vi "setPathAndType.vi"(8 "error in (no error)":errorcluster, 9 "fileType":T1, 10 "Path":path, 11 "reference in":refnum<class "excelFile.lvclass">) -> (0 "error out":errorcluster, 3 "reference out":refnum<class "excelFile.lvclass">)   [LabVIEW 2015, in "excelFile.lvclass"]
uses:
  excelFile.lvclass
  fileType.ctl
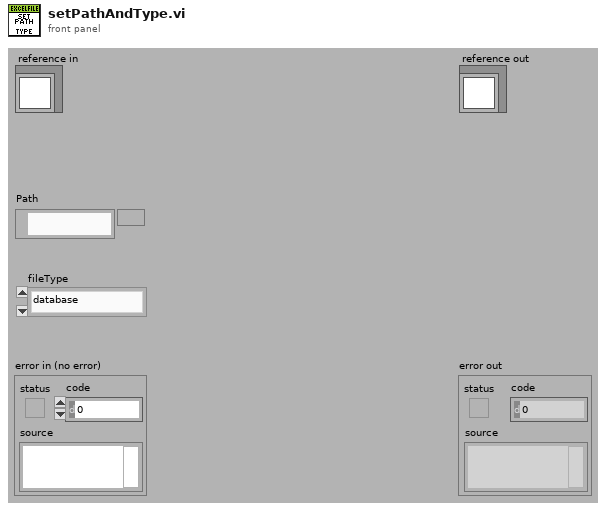
[diagram p1: front panel]
types:
  T1 = typedef "excelFile.lvclass/fileType.ctl" = enum16{"database", "CosmedTest"}
  T2 = typedef "excelFile.lvclass/ObjectAttributesRef.ctl" = refnum<data-value>
  T3 = typedef "excelFile.lvclass/ObjectAttributes.ctl" = cluster{"MyAttribute":dbl, "path":string, "Refnum Excel":cluster{"Excel._Application":refnum<k7>, "Workbooks":refnum<k7>, "Open":refnum<k7>}, "data":string[][][], "fileType":T1, "sheetName":string[]}
  T4 = typedef "excelFile.lvclass/ClassAttributesRef.ctl" = refnum<data-value>
  T5 = typedef "excelFile.lvclass/ClassAttributes.ctl" = cluster{"Dummy":bool, "excelFile_refs":refnum<class "excelFile.lvclass">[]}
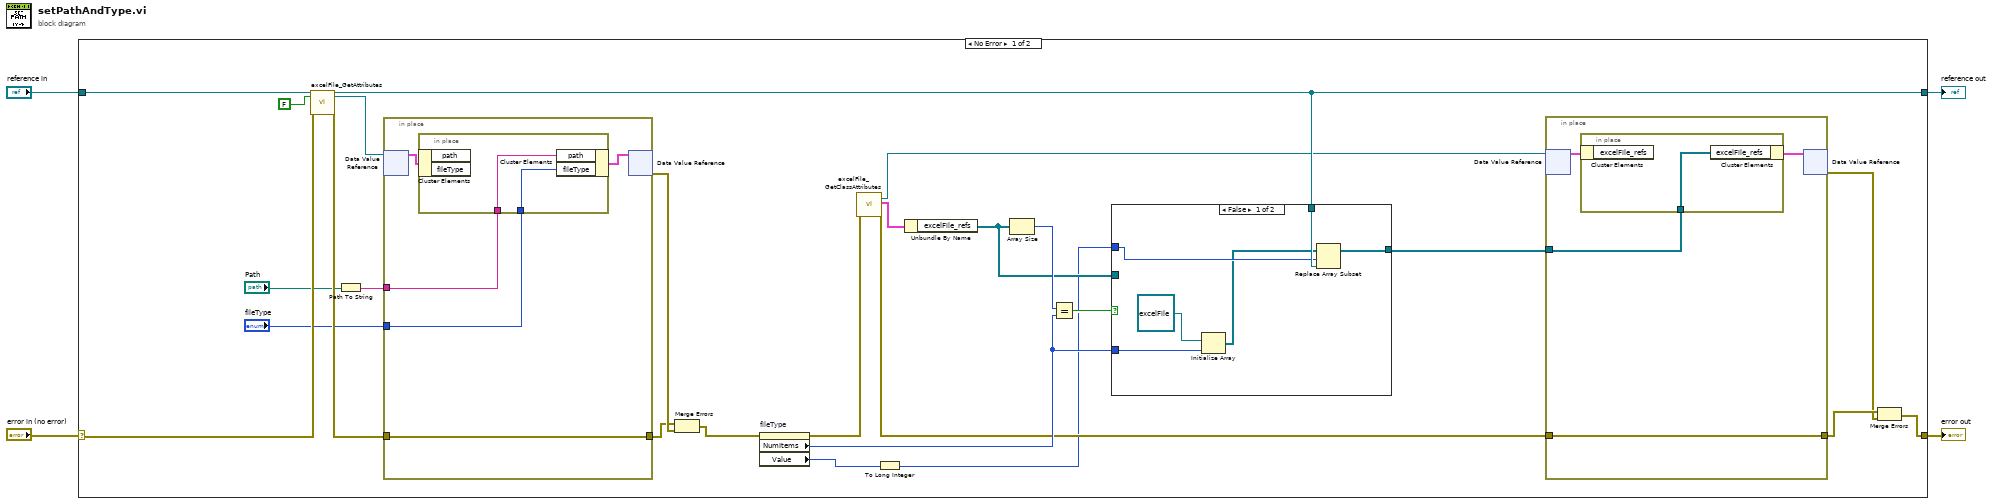
[diagram p0: block diagram]
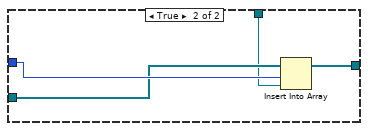
[diagram p2: hidden frame]
diagram:
  n1 = case shown="No Error" "error in (no error)" {
    selector: "error in (no error)" -> [w26 w54]
    tunnel: [w6 w54] -> w3
    tunnel: [w14 w53] -> w1
    tunnel: "reference in" -> [w28 w53]
    frame No Error {
      n2 = call "excelFile_GetAttributes.vi"("reference in"=w28, "return data? (T)"=FALSE, "error in (no error)"=w26) -> ("reference out"=w14:refnum<class "excelFile.lvclass">, "attributes ref"=w24:T2, "error out"=w25:errorcluster)  [unwired: 13 in, 1 out]
      n3 = Path To String(path="Path") -> (string=w22:string)
      n4 = in-place {
        in-place-border: w25 -> [w48]
        in-place-border: [w48] -> w29
        in-place-border: w22 -> [w47]
        in-place-border: "fileType" -> [w46]
        n5 = in-place-dvr #1(w24) -> (w49:T3)  [unwired: 1 out]
        n6 = in-place {
          in-place-border: w47 -> [w52]
          in-place-border: w46 -> [w51]
          n7 = in-place-cluster #2(w49) -> ()  [unwired: 2 out]
          n8 = in-place-cluster #2("path"=w52, "fileType"=w51) -> (w50:T3)
        }
        n9 = in-place-dvr #1(w50) -> (w30:errorcluster)  [unwired: 1 out]
      }
      n10 = Merge Errors(w29, w30) -> (w21:errorcluster)
      n11 = property on="fileType" class="Enum (strict)"(error in=w21) -> (error out=w20:errorcluster, "NumItems"=w15:u32, "Value"=w9:T1)  [unwired: 1 in, 1 out]
      n12 = call "excelFile_GetClassAttributes.vi"("error in (no error)"=w20) -> ("class attributes ref"=w11:T4, "class attributes"=w19:T5, "error out"=w12:errorcluster)  [unwired: 15 in, 1 out]
      n13 = To Long Integer(number=w9) -> (32bit integer=w8:i32)
      n14 = Unbundle By Name(w19) -> ("excelFile_refs"=w13:refnum<class "excelFile.lvclass">[])
      n15 = Array Size(array=w13) -> (size(s)=w18:i32)
      n16 = Equal?(x=w18, y=w15) -> (x = y?=w17:bool)
      n17 = case shown="False" w17 {
        tunnel: w8 -> [w38 w45]
        tunnel: w15 -> [w40 _]
        tunnel: w14 -> [w39 w43]
        tunnel: w13 -> [_ w44]
        tunnel: [w36 w42] -> w10
        frame False {
          n18 = Initialize Array(refnum<class "excelFile.lvclass"> refnum ("excelFile.lvclass"), w40) -> (w37:refnum<class "excelFile.lvclass">[])
          n19 = Replace Array Subset(array=w37, new element=w39, index=w38) -> (w36:refnum<class "excelFile.lvclass">[])
        }
        frame True {
          n20 = Insert Into Array(array=w44, index=w45, new element=w43) -> (w42:refnum<class "excelFile.lvclass">[])
        }
      }
      n21 = in-place {
        in-place-border: w12 -> [w32]
        in-place-border: [w32] -> w7
        in-place-border: w10 -> [w31]
        n22 = in-place-dvr #3(w11) -> (w33:T5)  [unwired: 1 out]
        n23 = in-place {
          in-place-border: w31 -> [w35]
          n24 = in-place-cluster #4(w33) -> ()  [unwired: 1 out]
          n25 = in-place-cluster #4("excelFile_refs"=w35) -> (w34:T5)
        }
        n26 = in-place-dvr #3(w34) -> (w5:errorcluster)  [unwired: 1 out]
      }
      n27 = Merge Errors(w7, w5) -> (w6:errorcluster)
    }
    frame Error {
    }
  }
  "error out" <- w3
  "reference out" <- w1
